vi "Sig_DO_Simple_Create.vi"(0 "reference in":refnum<class "Sig_DO_Simple.lvclass">, 5 "error in (no error)":errorcluster) -> (14 "reference out":refnum<class "Sig_DO_Simple.lvclass">, 19 "error out":errorcluster)   [LabVIEW 2019]
doc: "Constructor."
uses:
  <vilib>/addons/_AddQ/G#Object/G#Object.lvclass
  Sig_DO_Simple.lvclass
  D:/LabASF/LabASF/src/Signal_class/Signal.lvclass
  D:/LabASF/LabASF/src/Proccess_class/Proccess.lvclass
  Signal_class/Signal.lvclass
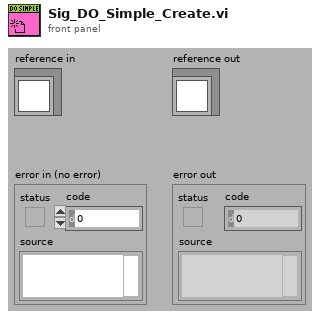
[diagram p1: front panel]
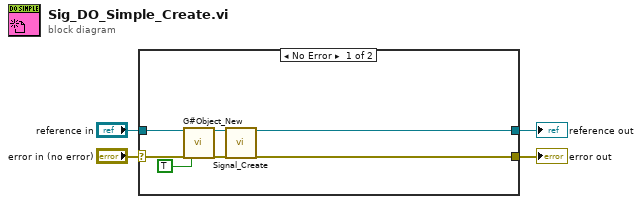
[diagram p0: block diagram]
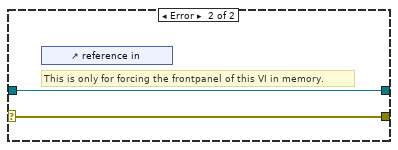
[diagram p2: hidden frame]
diagram:
  n1 = case shown="No Error" "error in (no error)" {
    selector: "error in (no error)" -> [w10 w13]
    tunnel: [w5 w13] -> w3
    tunnel: [w6 w12] -> w1
    tunnel: "reference in" -> [w11 w12]
    frame No Error {
      n2 = call <vilib>:"G#Object_New.vi"("reference in"=w11, "error in (no error)"=w10, "user counter (T)?"=TRUE ("User Counter")) -> ("reference out"=w8:refnum<class "G#Object.lvclass">, "error out"=w7:errorcluster)  [unwired: 14 in, 1 out]
      n3 = call "Signal_Create.vi"("reference in"=w8, "error in (no error)"=w7) -> ("reference out"=w6:refnum<class "Signal.lvclass">, "error out"=w5:errorcluster)  [unwired: 16 in]
    }
    frame Error {
      # "This is only for forcing the frontpanel of this VI in memory."
      n4 = control-ref of="reference in"() -> ()  [unwired: 1 out]
    }
  }
  "error out" <- w3
  "reference out" <- w1
